vi "TimedDialogZ.vi"(6 "dialog sec (60)":i32=60, 7 "options (0)":u16(ring) items=["continue", "retry", "end"], 8 "option list":string[](array[string])=["continue", "retry", "end"], 9 "Dialog text":string="Select an option and click ENTER") -> (2 "selection (timeout -1)":i32)   [LabVIEW 2016]
doc: "Displays a dialog message and a list of options for a user, and returns the user selection, or returns -1 if no user responds in a given time. A user should select an option and click Enter before the displayed time remaining reaches zero, or click on \"more time\". The \"options\" input sets the default user option, and the \"dialog sec\" input sets the initial time allowed (and the increment for \"more time\")."
panel:
  in  "More time":bool
  in  "pause (ms)":u32=100
  out "Time remaining (sec)":dbl format="%.2f"
  in  "Enter":bool
  out "error out":errorcluster
  in  "error in (no error)":errorcluster
  # "Program constants"
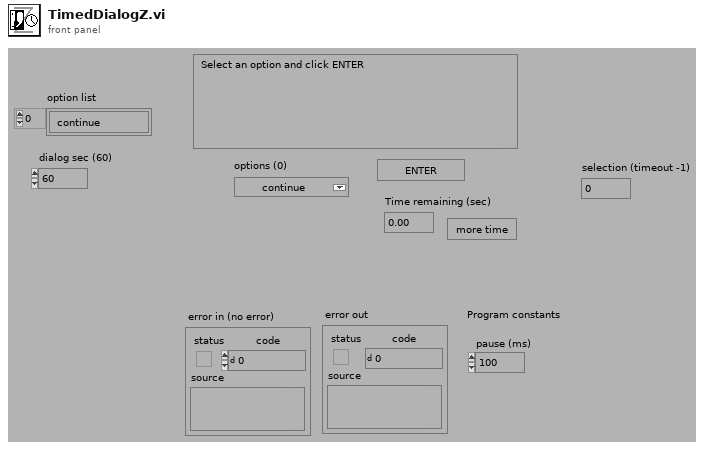
[diagram p1: front panel]
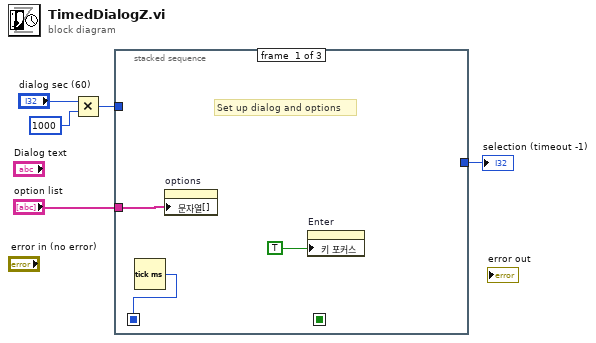
[diagram p0: block diagram]
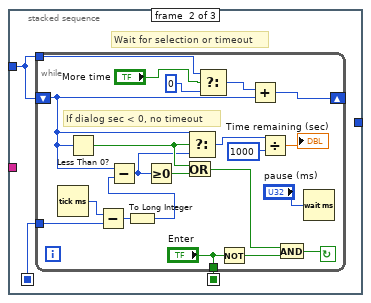
[diagram p2: hidden frame]
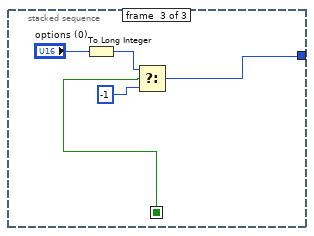
[diagram p3: hidden frame]
diagram:
  n1 = Multiply(x="dialog sec (60)", y=1000) -> (x*y=w2:i32)
  n2 = stacked-sequence {
    seq-local: [w7 _ _] -> [_ w11 _]
    seq-local: [_ w10 _] -> [_ _ w33]
    tunnel: "option list" -> [w8 _ _]
    tunnel: w2 -> [_ w9 _]
    tunnel: [_ _ w35] -> w4
    frame #0 {
      # "Set up dialog and options"
      n3 = Tick Count (ms)() -> (millisecond timer value=w7:u32)
      n4 = property on="options" class="Ring (엄격한)"("문자열[]"=w8) -> ()  [unwired: 2 in, 2 out]
      n5 = property on="Enter" class="Bool"("키 포커스"=TRUE ("Write Attribute")) -> ()  [unwired: 2 in, 2 out]
    }
    frame #1 {
      # "Wait for selection or timeout"
      n6 = while {
        tunnel: w9 -> [w17]
        shift-left: w9 -> [w12]
        shift-right: [w13] -> _
        tunnel: ["Enter"] -> w10
        tunnel: w11 -> [w31]
        stop <- w25 continue-if-true
        # "If dialog sec < 0, no timeout"
        n7 = Tick Count (ms)() -> (millisecond timer value=w32:u32)
        n8 = Less Than 0?(x=w12) -> (x < 0?=w24:bool)
        n9 = Subtract(x=w32, y=w31) -> (x-y=w30:u32)
        n10 = To Long Integer(number=w30) -> (32bit integer=w29:i32)
        n11 = Subtract(x=w12, y=w29) -> (x-y=w23:i32)
        n12 = Greater Or Equal To 0?(x=w23) -> (x >= 0?=w28:bool)
        n13 = Or(x=w24, y=w28) -> (x .or. y?=w26:bool)
        n14 = Select(t=w12, s=w24, f=w23) -> (s? t:f=w21:i32)
        n15 = Select(t=w17, s="More time", f=0) -> (s? t:f=w14:i32)
        n16 = Not(x="Enter") -> (.not. x?=w27:bool)
        n17 = Add(x=w14, y=w12) -> (x+y=w13:i32)
        n18 = Divide(x=w21, y=1000) -> (x/y=→"Time remaining (sec)":dbl)
        n19 = And(x=w26, y=w27) -> (x .and. y?=w25:bool)
        n20 = Wait (ms)(milliseconds to wait="pause (ms)") -> ()  [unwired: 1 out]
      }
    }
    frame #2 {
      n21 = To Long Integer(number="options (0)") -> (32bit integer=w36:i32)
      n22 = Select(t=w36, s=w33, f=-1) -> (s? t:f=w35:i32)
    }
  }
  "selection (timeout -1)" <- w4
